vi "String Functions 2a.vi"() -> ()   [LabVIEW 2015]
panel:
  out "Welcome Message":string
  in  "User Name":string
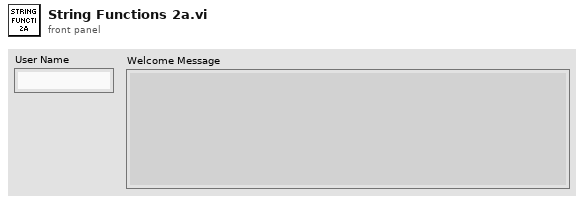
[diagram p1: front panel]
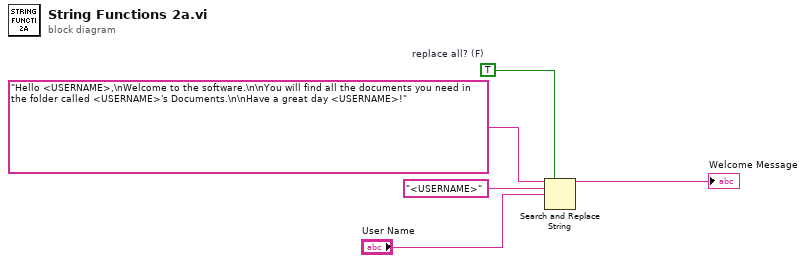
[diagram p0: block diagram]
diagram:
  w2 = TRUE  # replace all? (F)
  n1 = Search and Replace String(replace all?=w2, input string="Hello <USERNAME>,\nWelcome to the software.\n\nYou will find all the documents you need in the folder called <USERNAME>'s Documents.\n\nHave a great day <USERNAME>!", search string="<USERNAME>", replace string="User Name") -> (result string=→"Welcome Message":string)  [unwired: 4 in, 3 out]
